vi "Packet Number.vi"(8 "Error In":errorcluster, 10 "Action":T5, 11 "LINX Device Config":T1) -> (0 "Error Out":errorcluster, 2 "Packet Number":u16, 3 "LINX Device Config":T1)   [LabVIEW 2020, in "LMH-LINX.lvlib" / "Device.lvlib"]
doc: "FGV to store the current packet number.\n\nInitialize sets the current packet number to 0.\nGet returns the current packet number.\nIncrement increments the current packet number and returns the new packet number."
uses:
  Device.lvlib
  Type Defs/Packet Number FGV Action.ctl
  Type Defs/LINX Device Config.ctl
  Type Defs/Interface.ctl
  Type Defs/TCP Config.ctl
  Type Defs/Channels.ctl
  LMH-LINX.lvlib
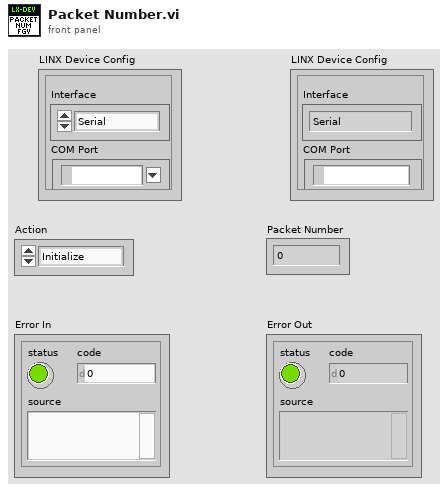
[diagram p1: front panel]
types:
  T1 = typedef "LMH-LINX.lvlib/Device.lvlib/LINX Device Config.ctl" = cluster{"Interface":T2, "COM Port":refnum<visa-resource-name>, "TCP Configuration":T3, "Device Family":u8, "Device ID":u8, "Device Name":string, "TCP Ref":refnum<k5>, "Channels":T4}
  T2 = typedef "LMH-LINX.lvlib/Interface.ctl" = enum16{"Serial", "TCP"}
  T3 = typedef "LMH-LINX.lvlib/Device.lvlib/TCP Config.ctl" = cluster{"IP Address":string, "Port":u16}
  T4 = typedef "LMH-LINX.lvlib/Channels.ctl" = cluster{"DI":u8[], "DO":u8[], "AI":u8[], "AO":u8[], "PWM":u8[], "QE":u8[], "UART":u8[], "I2C 2":u8[], "SPI":u8[], "CAN":u8[], "Servo":u8[], "AI Ref (V)":dbl, "AI Resolution (Bits)":u8, "AO Ref (V)":dbl, "AO Resolution (Bits)":u8}
  T5 = typedef "LMH-LINX.lvlib/Device.lvlib/Packet Number FGV Action.ctl" = enum16{"Initialize", "Get", "Increment"}
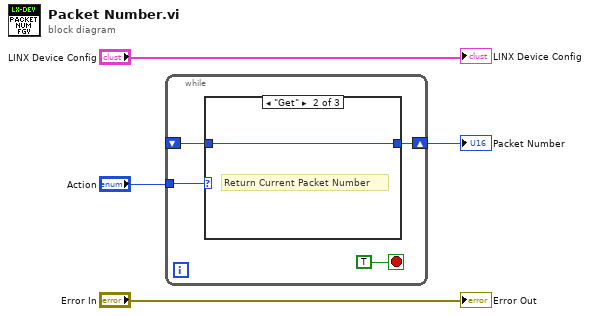
[diagram p0: block diagram]
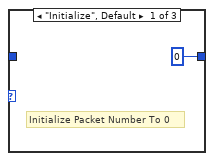
[diagram p2: hidden frame]
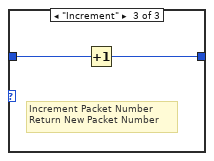
[diagram p3: hidden frame]
diagram:
  n1 = while {
    tunnel: "Action" -> [w7]
    shift-right: [w5] -> w3
    shift-left: _ -> [w6]
    stop <- TRUE stop-if-true
    n2 = case shown="\"Get\"" w7 {
      tunnel: w6 -> [_ w10 w12]
      tunnel: [u16 0 ("Numeric Control") w10 w11] -> w5
      frame "Initialize", Default {
        # "Initialize Packet Number To 0"
      }
      frame "Get" {
        # "Return Current Packet Number"
      }
      frame "Increment" {
        # "Increment Packet Number\nReturn New Packet Number"
        n3 = Increment(x=w12) -> (x+1=w11:u16)
      }
    }
  }
  "Packet Number" <- w3
  "LINX Device Config" <- "LINX Device Config"
  "Error Out" <- "Error In"
